vi "Set Setting.vi"(7 "Depth":T3 items=["WRITE AREA", "RUNNING AREA", "SAVE AREA"], 8 "error in (no error)":errorcluster, 9 "Setting Data":u8[](array[numeric]), 10 "Target Setting":T1={"Type"=1, "Category"=0, "Item"=0, "Target 1"=0, "Target 2"=0, "Target 3"=0, "Target 4"=0} {"Type" items=["ENVIRONMENT"=1, "COMMON MEASUREMENT"=2, "PROGRAM 0"=16, "PROGRAM 1"=17, "PROGRAM 2"=18, "PROGRAM 3"=19, "PROGRAM 4"=20, "PROGRAM 5"=21, "PROGRAM 6"=22, "PROGRAM 7"=23, "PROGRAM 8"=24, "PROGRAM 9"=25, "PROGRAM 10"=26, "PROGRAM 11"=27, "PROGRAM 12"=28, "PROGRAM 13"=29, "PROGRAM 14"=30, "PROGRAM 15"=31]}, 11 "Device ID (0)":i32) -> (0 "error out":errorcluster, 2 "Setting Error":u32, 3 "Device ID out":i32)   [LabVIEW 2014, in "Keyence LJ-V7000.lvlib"]
doc: "This function sends the setting for the specified item to the controller.\n\n<B>Note</B>: \nFor the procedure to reflect the setting on the controller, see <B>9.3</B> in a manual of measuring instrument drivers."
uses:
  Keyence LJ-V7000.lvlib
  constant/Setting Depth.ctl
  Clusters/Target Setting.ctl
  constant/Setting Type.ctl
  constant/Driver VI No.ctl
panel:
  # "(c) 2012 KEYENCE CORPORATION.  ALL RIGHTS RESERVED."
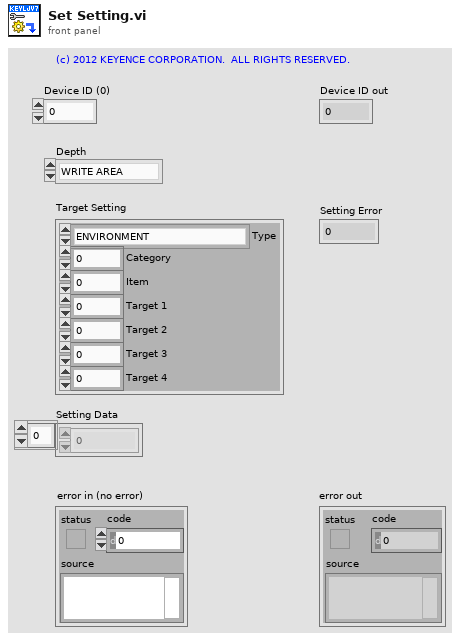
[diagram p1: front panel]
types:
  T1 = typedef "Keyence LJ-V7000.lvlib/Target Setting.ctl" = cluster{"Type":T2, "Category":u8, "Item":u8, "Target 1":u8, "Target 2":u8, "Target 3":u8, "Target 4":u8}
  T2 = typedef "Keyence LJ-V7000.lvlib/Setting Type.ctl" = u8
  T3 = typedef "Keyence LJ-V7000.lvlib/Setting Depth.ctl" = u8
  T4 = typedef "Keyence LJ-V7000.lvlib/Driver VI No.ctl" = enum16{"Initialize", "Close", "Reboot Controller", "Return to Factory State", "Get System Error", "Clear System Error", "Trigger", "Start Batch Measurements", "Stop Batch Measurements", "Auto Zero", "Timing", "Reset", "Clear Memory", "Set Setting", "Get Setting", "Initialize Setting", "Reflect Setting", "Update Write Settings Area", "Check Status of Saving to Save Area", "Set Time", "Get Time", "Change Program", "Read Active Program Number", "Read Measurement Data", "Read Profiles(for High-Speed Mode)", "Read Batch Profiles(for High-Speed Mode)", "Read Profiles(for Advanced Mode)", "Read Batch Profiles(for Advanced Mode)", "Start Storage", "Stop Storage", "Read Storage Status", "Read Data Storage Data", "Read Profile Storage Data", "Read Batch Profile Storage Data", "Start High-Speed Data Communication", "Stop High-Speed Data Communication", "Read Profiles(for High-Speed Communication)"}
  T5 = cluster{"Type":T2, "Category":u8, "Item":u8, "reserve":u8, "Target 1":u8, "Target 2":u8, "Target 3":u8, "Target 4":u8}
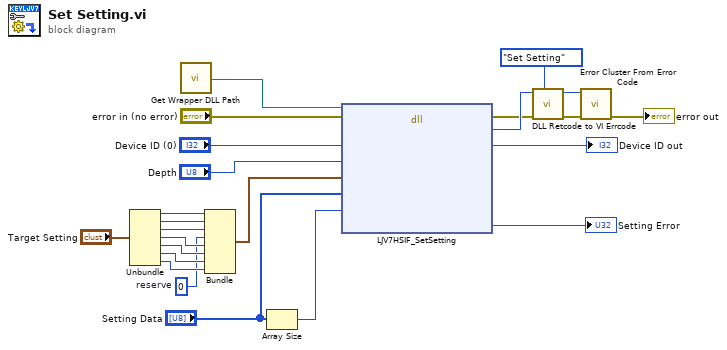
[diagram p0: block diagram]
diagram:
  w12 = u8 0  # reserve
  n1 = Unbundle("Target Setting") -> ("Type"=w19:T2, "Category"=w18:u8, "Item"=w17:u8, "Target 1"=w16:u8, "Target 2"=w15:u8, "Target 3"=w14:u8, "Target 4"=w13:u8)
  n2 = call "Get Wrapper DLL Path.vi"() -> ("Wrapper DLL Path"=w7:path)  [unwired: 1 in]
  n3 = Bundle("Type"=w19, "Category"=w18, "Item"=w17, "reserve"=w12, "Target 1"=w16, "Target 2"=w15, "Target 3"=w14, "Target 4"=w13) -> (w11:T5)  [unwired: 1 in]
  n4 = Array Size(array="Setting Data") -> (size(s)=w9:i32)
  n5 = dll-call lib="C:/Program Files/National Instruments/LabVIEW 2011/instr.lib/Keyence LJ-V7000/LJV7_HighSpeedWrapper.dll" fn="LJV7HSIF_SetSetting"(path in=w7, error in="error in (no error)", "lDeviceId"="Device ID (0)", "byDepth"="Depth", "pTargetSetting"=w11, "pData"="Setting Data", "dwDataSize"=w9) -> (error out=w3:errorcluster, "lRetCode"=w4:i32, "lDeviceId"=→"Device ID out":i32, "pdwError"=→"Setting Error":u32)  [unwired: 6 in, 1 out]
  n6 = call "DLL Retcode to VI Errcode.vi"("Driver VI No"=Driver_VI_No."Set Setting", "error in (no error)"=w3, "DLL Return Code"=w4) -> ("error out"=w6:errorcluster, "VI Error Code"=w5:i32)  [unwired: 7 in]
  n7 = call <vilib>:"Error Cluster From Error Code.vi"("error in (no error)"=w6, "error code (0)"=w5) -> ("error out"=→"error out":errorcluster)  [unwired: 7 in]
